vi "Update Lists.vi"(8 "error in (no error)":errorcluster, 11 "Fault Monitor in":refnum<class "Fault Monitor.lvclass">) -> (0 "error out":errorcluster, 3 "Fault Monitor out":refnum<class "Fault Monitor.lvclass">)   [LabVIEW 2023, in "Fault Monitor.lvlib" / "Fault Monitor.lvclass"]
uses:
  Library/Fault Monitor.lvclass
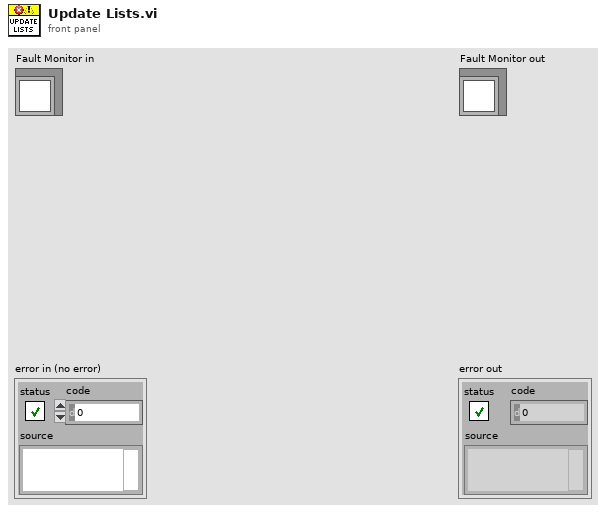
[diagram p1: front panel]
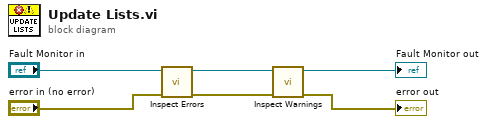
[diagram p0: block diagram]
diagram:
  n1 = call "Inspect Errors.vi"("error in (no error)"="error in (no error)", "Fault Monitor in"="Fault Monitor in") -> ("error out"=w3:errorcluster, "Fault Monitor out"=w6:refnum<class "Fault Monitor.lvclass">)  [unwired: 8 in]
  n2 = call "Inspect Warnings.vi"("error in (no error)"=w3, "Fault Monitor in"=w6) -> ("error out"=→"error out":errorcluster, "Fault Monitor out"=→"Fault Monitor out":refnum<class "Fault Monitor.lvclass">)  [unwired: 8 in]
